vi "Snap.vi"(8 "error in (no error)":errorcluster, 11 "CameraDemo in":refnum<class "CameraDemo.lvclass">) -> (0 "error out":errorcluster, 2 "SnapInfo":T1, 3 "CameraDemo out":refnum<class "CameraDemo.lvclass">)   [LabVIEW 2020, in "CameraI2COUSB.lvlib" / "CameraDemo.lvclass"]
uses:
  CameraDemo.lvclass
  CameraDemo.lvclass/CameraDemo.ctl
  ICamera/ICamera/TypeDef/SnapInfo.ctl
  ICamera/ICamera/ICamera.lvclass
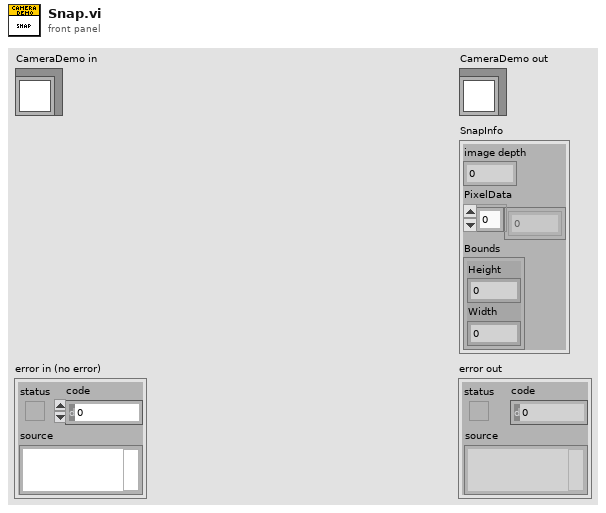
[diagram p1: front panel]
types:
  T1 = typedef "ICamera.lvlib/ICamera.lvclass/SnapInfo.ctl" = cluster{"image depth":i32, "PixelData":u8[], "Bounds":cluster{"Height":i16, "Width":i16}}
  T2 = typedef "imagedata.ctl" = cluster{"image type":i32, "image depth":i32, "image":u8[], "mask":u8[], "colors":u32[], "Rectangle":cluster{"left":i16, "top":i16, "right":i16, "bottom":i16}}
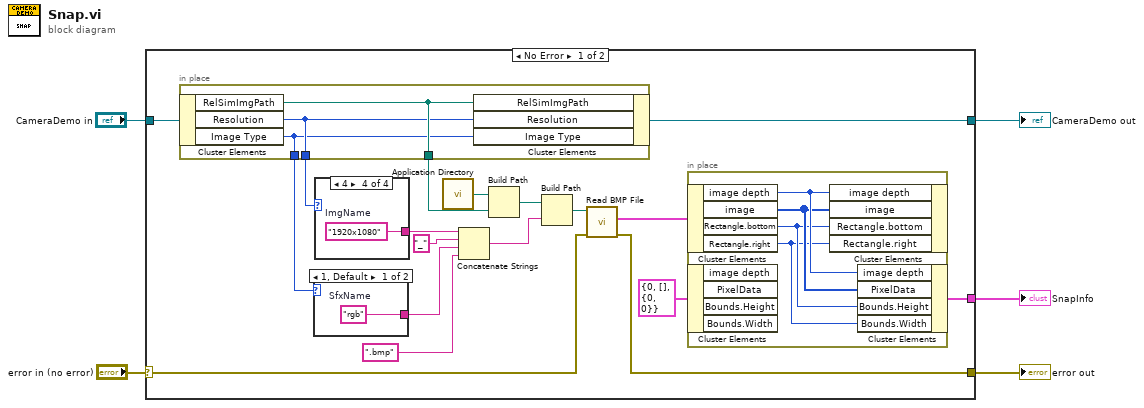
[diagram p0: block diagram]
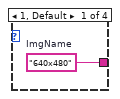
[diagram p2: hidden frame]
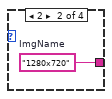
[diagram p3: hidden frame]
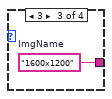
[diagram p4: hidden frame]
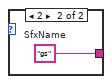
[diagram p5: hidden frame]
diagram:
  n1 = case shown="No Error" "error in (no error)" {
    selector: "error in (no error)" -> [w7 w38]
    tunnel: "CameraDemo in" -> [w23 w37]
    tunnel: [w22 w37] -> w3
    tunnel: [w8 _] -> w2
    tunnel: [w6 w38] -> w1
    frame No Error {
      n2 = in-place {
        in-place-border: [w36] -> w14
        in-place-border: [w35] -> w13
        in-place-border: [w34] -> w12
        n3 = in-place-cluster #1(w23) -> ("RelSimImgPath"=w36:path, "Resolution"=w35:u8, "Image Type"=w34:u8)
        n4 = in-place-cluster #1("RelSimImgPath"=w36, "Resolution"=w35, "Image Type"=w34) -> (w22:refnum<class "CameraDemo.lvclass">)
      }
      n5 = case shown="1, Default" w12 {
        tunnel: [w32 w33] -> w20
        frame 1, Default {
          w32 = "rgb"  # SfxName
        }
        frame 2 {
          w33 = "gs"  # SfxName
        }
      }
      n6 = case shown="4" w13 {
        tunnel: [w28 w29 w30 w31] -> w19
        frame 1, Default {
          w28 = "640x480"  # ImgName
        }
        frame 2 {
          w29 = "1280x720"  # ImgName
        }
        frame 3 {
          w30 = "1600x1200"  # ImgName
        }
        frame 4 {
          w31 = "1920x1080"  # ImgName
        }
      }
      n7 = call <vilib>:"Application Directory.vi"() -> ("Application Directory"=w18:path)
      n8 = Concatenate Strings(w19, "_" ("string"), w20, ".bmp" ("string")) -> (w21:string)
      n9 = Build Path(base path=w18, name or relative path=w14) -> (appended path=w17:path)
      n10 = Build Path(base path=w17, name or relative path=w21) -> (appended path=w11:path)
      n11 = call <vilib>:"Read BMP File.vi"("error in (no error)"=w7, "path to BMP file"=w11) -> ("error out"=w6:errorcluster, "image data"=w10:T2)  [unwired: 7 in, 1 out]
      n12 = in-place {
        n13 = in-place-cluster #2(w10) -> ("image depth"=w27:i32, "image"=w26:u8[], "Rectangle.bottom"=w25:i16, "Rectangle.right"=w24:i16)
        n14 = in-place-cluster #3(T1 {"image depth"=0, "PixelData"=[], "Bounds"={"Height"=0, "Width"=0}} ("SnapInfo")) -> ()  [unwired: 4 out]
        n15 = in-place-cluster #2("image depth"=w27, "image"=w26, "Rectangle.bottom"=w25, "Rectangle.right"=w24) -> ()  [unwired: 1 out]
        n16 = in-place-cluster #3("image depth"=w27, "PixelData"=w26, "Bounds.Height"=w25, "Bounds.Width"=w24) -> (w8:T1)
      }
    }
    frame Error {
    }
  }
  "CameraDemo out" <- w3
  "SnapInfo" <- w2
  "error out" <- w1
